vi "autoGetIOData.vi"(11 "elapsed auton time":dbl) -> (3 "sensor datas":T2)   [LabVIEW 2012]
panel:
  out "output cluster":T1
  in  "const":T2
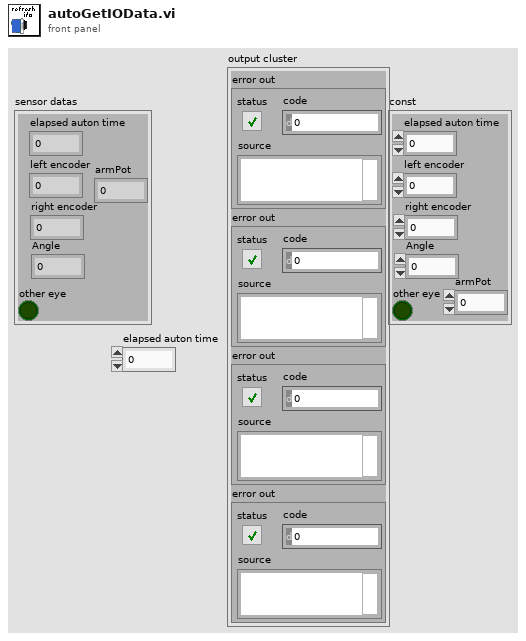
[diagram p1: front panel]
types:
  T1 = cluster{"error out":errorcluster, "error out":errorcluster, "error out":errorcluster, "error out":errorcluster}
  T2 = cluster{"elapsed auton time":dbl, "left encoder":dbl, "other eye":bool, "right encoder":dbl, "Angle":dbl, "armPot":dbl}
  T3 = typedef "WPI_AnalogChannelDevRef.ctl" = cluster{"DevStatus":errorcluster, "Analog Module":T4, "Analog Channel":T5}
  T4 = typedef "FPGA_TypedefAnalogModule.ctl" = enum16{"Analog Module 1", "Analog Module 2"}
  T5 = typedef "FPGA_AIChannel.ctl" = enum8{"AI 1", "AI 2", "AI 3", "AI 4", "AI 5", "AI 6", "AI 7", "AI 8", "Invalid"}
  T6 = typedef "WPI_GyroDevRef.ctl" = cluster{"DevStatus":errorcluster, "Analog Module":T4, "Analog Channel":T5, "Offset":dbl, "Gain (VoltsPerDegree/Second)":dbl}
  T7 = typedef "WPI_EncoderDevRef.ctl" = cluster{"DevStatus":errorcluster, "EncoderIndex":T8, "CounterIndex":T9, "DistancePerCount":dbl, "Decoding Type":T10}
  T8 = typedef "FPGA_EncoderIdx.ctl" = enum8{"Enc 0", "Enc 1", "Enc 2", "Enc 3", "Invalid"}
  T9 = typedef "FPGA_CounterCtrSystemIndex.ctl" = enum8{"Ctr 0", "Ctr 1", "Ctr 2", "Ctr 3", "Ctr 4", "Ctr 5", "Ctr 6", "Ctr 7", "Invalid"}
  T10 = typedef "WPI_EncoderType.ctl" = enum16{"1x", "2x", "4x"}
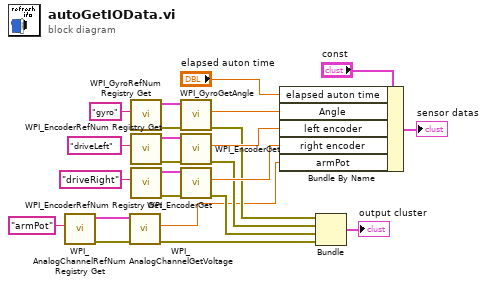
[diagram p0: block diagram]
diagram:
  n1 = call <vilib>:"WPI_AnalogChannelRefNum Registry Get.vi"("refnum name"="armPot") -> ("error out"=w4:errorcluster, "AIDeviceRef"=w7:T3)  [unwired: 9 in]
  n2 = call <vilib>:"WPI_AnalogChannelGetVoltage.vi"("error in (no error)"=w4, "AIDeviceRef"=w7) -> ("error out"=w3:errorcluster, "Voltage"=w5:dbl)  [unwired: 7 in, 1 out]
  n3 = call <vilib>:"WPI_GyroRefNum Registry Get.vi"("refnum name"="gyro") -> ("error out"=w9:errorcluster, "GyroDevRef"=w10:T6)  [unwired: 9 in]
  n4 = call <vilib>:"WPI_EncoderRefNum Registry Get.vi"("refnum name"="driveLeft") -> ("error out"=w15:errorcluster, "EncoderDevRef"=w16:T7)  [unwired: 9 in]
  n5 = call <vilib>:"WPI_EncoderRefNum Registry Get.vi"("refnum name"="driveRight") -> ("error out"=w12:errorcluster, "EncoderDevRef"=w11:T7)  [unwired: 9 in]
  n6 = call <vilib>:"WPI_GyroGetAngle.vi"("error in (no error)"=w9, "GyroDevRef"=w10) -> ("error out"=w19:errorcluster, "Angle"=w22:dbl)  [unwired: 6 in, 2 out]
  n7 = call <vilib>:"WPI_EncoderGet.vi"("error in (no error)"=w15, "EncoderDevRef"=w16) -> ("error out"=w18:errorcluster, "Distance"=w21:dbl)  [unwired: 4 in, 4 out]
  n8 = call <vilib>:"WPI_EncoderGet.vi"("error in (no error)"=w12, "EncoderDevRef"=w11) -> ("error out"=w17:errorcluster, "Distance"=w20:dbl)  [unwired: 4 in, 4 out]
  n9 = Bundle By Name(cluster="const", "elapsed auton time"="elapsed auton time", "Angle"=w22, "left encoder"=w21, "right encoder"=w20, "armPot"=w5) -> (→"sensor datas":T2)
  n10 = Bundle("error out"=w19, "error out"=w18, "error out"=w17, "error out"=w3) -> (→"output cluster":T1)  [unwired: 1 in]
